vi "Expt_5_Transmitter_Demo.vi"() -> ()   [LabVIEW 2022 SP3]
uses:
  <vilib>/Analysis/NI_AALPro.lvlib
  <vilib>/measure/NI_MABase.lvlib
panel:
  out "Waveform Chart 2":waveform(dbl)[](graph)
  out "XY Graph":cluster{i32[], i32[]}(graph)
  out "Array 2":i32[](array[numeric])
  out "Array":i32[](array[numeric])
  in  "User Input For Iterations":i32
  out "Numeric":dbl
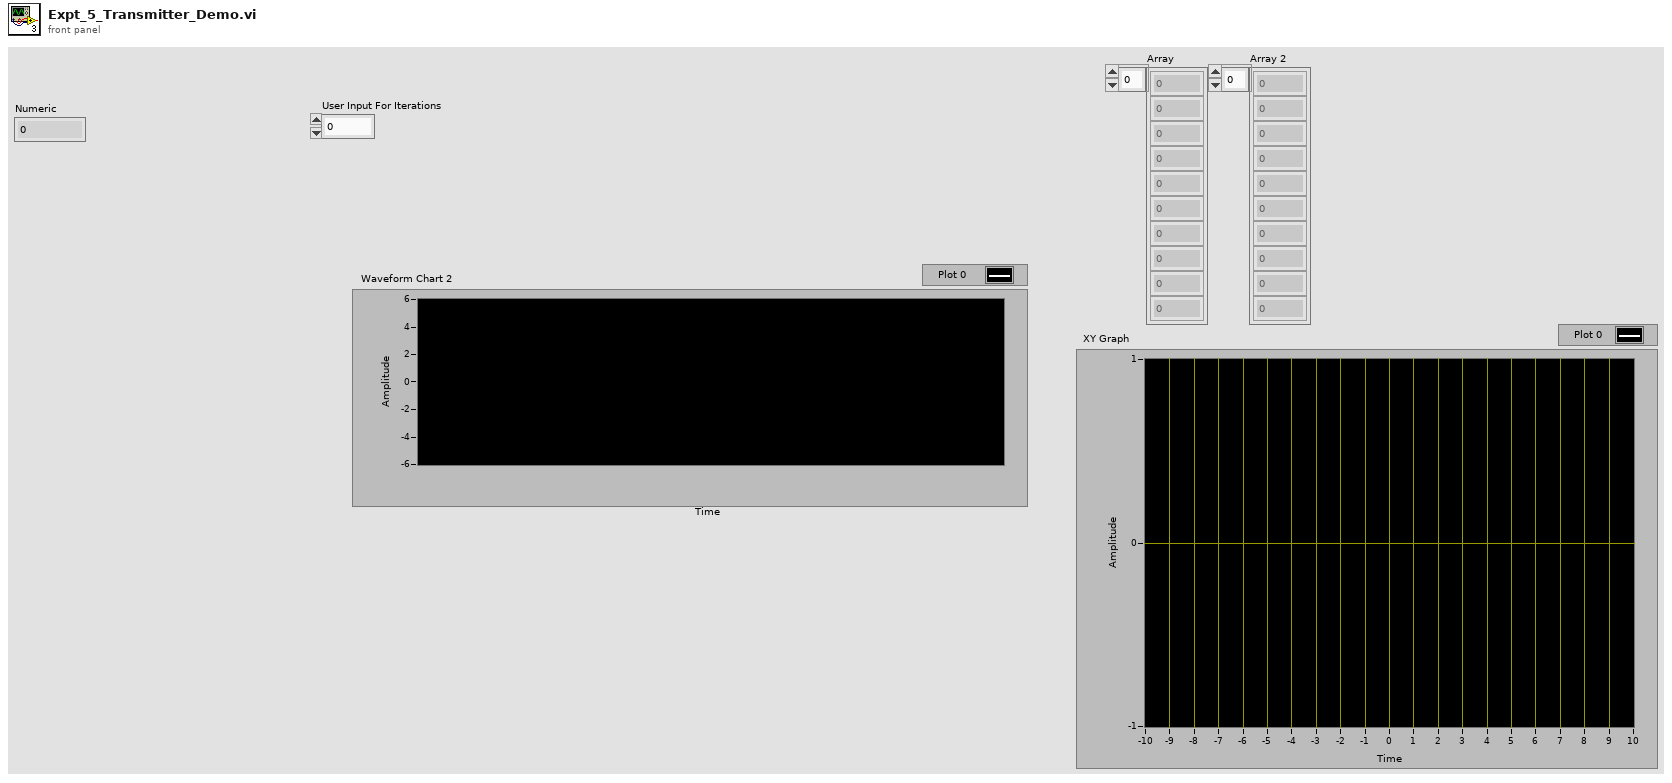
[diagram p1: front panel]
types:
  T1 = enum16{"sine", "cosine", "triangle", "square", "sawtooth", "increasing ramp", "decreasing ramp"}
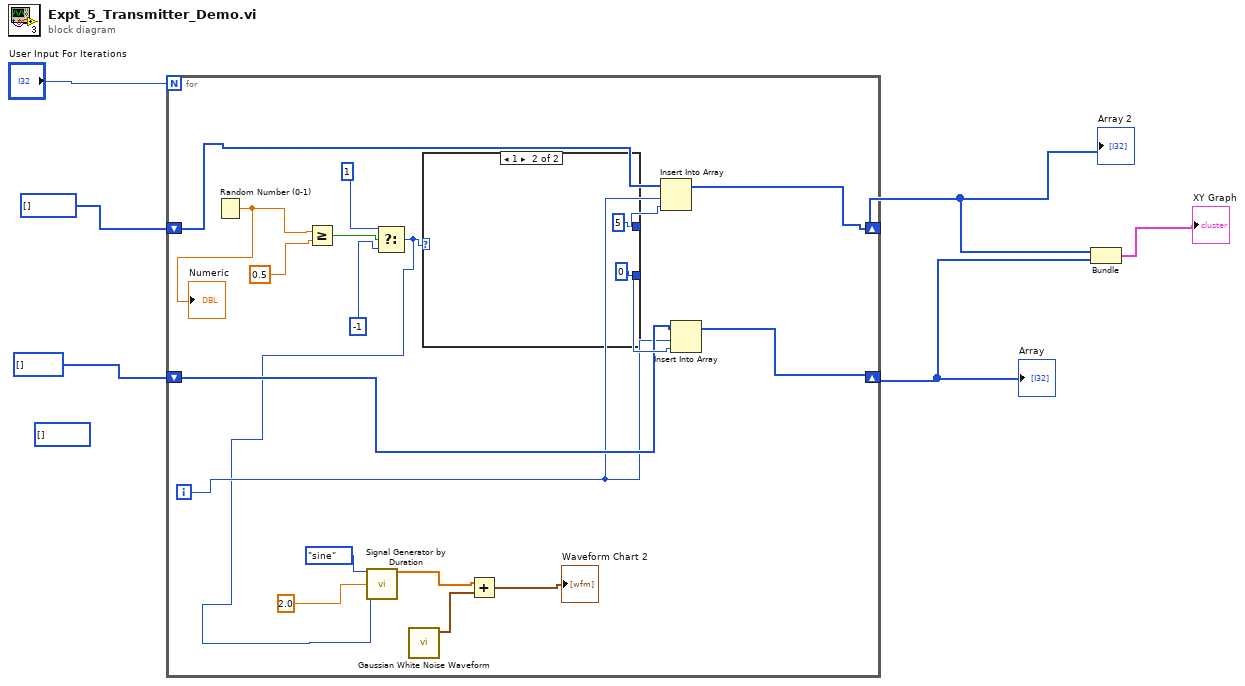
[diagram p0: block diagram]
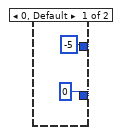
[diagram p2: hidden frame]
diagram:
  (unwired) i32[] []
  n1 = for {
    N: "User Input For Iterations" -> [_]
    shift-right: [w16] -> w3
    shift-left: i32[] [] -> [w18]
    shift-right: [w15] -> w2
    shift-left: i32[] [] -> [w17]
    i -> [w13]
    n2 = Random Number (0-1)() -> (number: 0 to 1=w14:dbl)
    "Numeric" <- w14
    n3 = Greater Or Equal?(x=w14, y=0.5) -> (x >= y?=w23:bool)
    n4 = Select(t=1, s=w23, f=-1) -> (s? t:f=w10:i32)
    n5 = call <vilib>:"Signal Generator by Duration.vi"("signal type"=T1."sine", "frequency"=2.0, "amplitude"=w10) -> ("signal"=w9:dbl[])  [unwired: 9 in, 3 out]
    n6 = call <vilib>:"Gaussian White Noise Waveform.vi"() -> ("signal out"=w8:waveform(dbl))  [unwired: 10 in, 1 out]
    n7 = case shown="1" w10 {
      tunnel: [-5 5] -> w20
      tunnel: [0 0] -> w19
      frame 0, Default {
      }
      frame 1 {
      }
    }
    n8 = Add(x=w9, y=w8) -> (x+y=→"Waveform Chart 2":waveform(dbl)[])
    n9 = Insert Into Array(array=w18, index=w13, new element=w20) -> (w16:i32[])
    n10 = Insert Into Array(array=w17, index=w13, new element=w19) -> (w15:i32[])
  }
  "Array" <- w2
  "Array 2" <- w3
  n11 = Bundle(w3, w2) -> (→"XY Graph":cluster{i32[], i32[]})  [unwired: 1 in]
